vi "Close MeasurementLink Session.vi"(8 "error in":errorcluster, 9 "initialize and close session behavior":T1, 10 "session in":variant, 11 "session factory in":refnum<class "Session Factory.lvclass">) -> (0 "error out":errorcluster)   [LabVIEW 2021, in "Session Management niDAQmx.lvlib" / "Session Factory.lvclass"]
doc: "Closes the local session. If the session represents a remote session, <b>initialize and close session behavior</b> determines whether closing the local session closes the server session or detaches from the server session."
uses:
  Session Factory.lvclass
  <vilib>/Plug-In SDKs/Sessions/Instrument/ISession Factory/Initialize and Close Session Behavior.ctl
  Session Factory.lvclass/Session Factory.ctl
  NI_DAQmx_client/RPC Messages/nidaqmx_grpc_ClearTaskRequest.ctl
  NI_DAQmx_client/RPC Messages/nidevice_grpc_Session.ctl
  NI_DAQmx_client/RPC Messages/nidevice_grpc_Session_session/nidevice_grpc_Session_session.lvclass
  NI_DAQmx_client/NI_DAQmx_client.lvlib
  <vilib>/Plug-In SDKs/Sessions/Instrument/ISession Factory/ISession Factory.lvclass
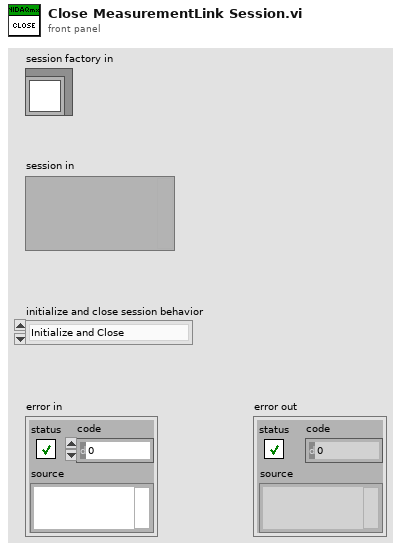
[diagram p1: front panel]
types:
  T1 = typedef "NI Session Management Instrument.lvlib/ISession Factory.lvclass/Initialize and Close Session Behavior.ctl" = enum16{"Initialize and Close", "Attach and Detach", "Initialize and Detach", "Attach and Close"}
  T2 = typedef "NI_DAQmx_client.lvlib/nidaqmx_grpc_ClearTaskRequest.ctl" = cluster{"task":T3}
  T3 = typedef "NI_DAQmx_client.lvlib/nidevice_grpc_Session.ctl" = cluster{"nidevice_grpc_Session_session":refnum<class "nidevice_grpc_Session_session.lvclass">}
  T4 = typedef "grpc-lvsupport-release.lvlib/grpcId.ctl" = u64
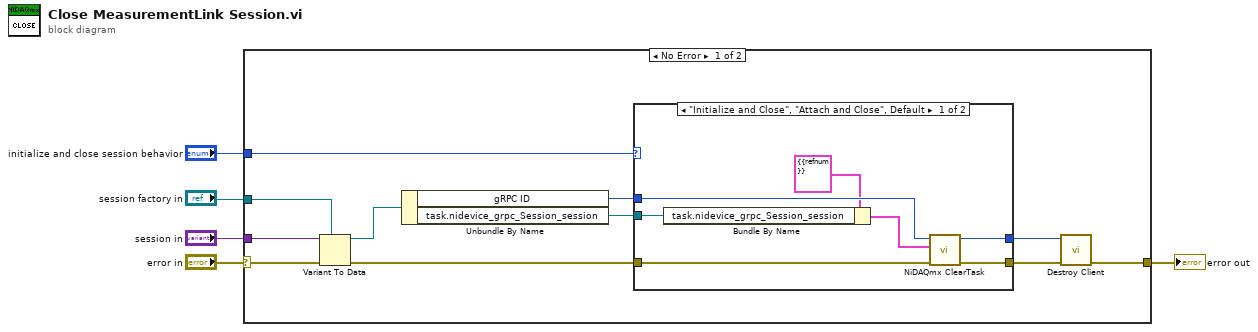
[diagram p0: block diagram]
diagram:
  n1 = case shown="No Error" "error in" {
    selector: "error in" -> [w10 w26]
    tunnel: [w11 w26] -> w4
    tunnel: "session factory in" -> [w7 _]
    tunnel: "session in" -> [w8 _]
    tunnel: "initialize and close session behavior" -> [w14 _]
    frame No Error {
      n2 = Variant To Data(error in=w10, type=w7, Variant=w8) -> (data=w6:refnum<class "Session Factory.lvclass">, error out=w9:errorcluster)
      n3 = Unbundle By Name(w6) -> ("gRPC ID"=w16:T4, "task.nidevice_grpc_Session_session"=w15:refnum<class "nidevice_grpc_Session_session.lvclass">)
      n4 = case shown="\"Initialize and Close\", \"Attach and Close\", Default" w14 {
        tunnel: w9 -> [w23 w24]
        tunnel: [w22 w24] -> w12
        tunnel: w16 -> [w21 w25]
        tunnel: w15 -> [w19 _]
        tunnel: [w17 w25] -> w13
        frame "Initialize and Close", "Attach and Close", Default {
          n5 = Bundle By Name(cluster=T2 {"task"={"nidevice_grpc_Session_session"=refnum}} ("Request Data"), "task.nidevice_grpc_Session_session"=w19) -> (w18:T2)
          n6 = call "NiDAQmx ClearTask.vi"("error in"=w23, "Request Data"=w18, "gRPC ID"=w21) -> ("error out"=w22:errorcluster, "gRPC ID out"=w17:T4)  [unwired: 6 in, 1 out]
        }
        frame "Attach and Detach", "Initialize and Detach" {
        }
      }
      n7 = call "Destroy Client.vi"("error in"=w12, "gRPC ID"=w13) -> ("error out"=w11:errorcluster)  [unwired: 9 in]
    }
    frame Error {
    }
  }
  "error out" <- w4
